vi "Release Session.vi"(6 "force destroy? (F)":bool, 8 "error in":errorcluster, 11 "Session Handle":T1) -> (0 "error out":errorcluster, 3 "file path":path)   [LabVIEW 2015, in "Config Data.lvclass"]
doc: "Release the configuration session for the given reference. If this is the last reference to return, then the config data file will be closed and the file path for the configuration file will be returned."
uses:
  Config Data.lvclass
  Config Session.ctl
  <userlib>/_Session Fwk/Session - Root.lvclass
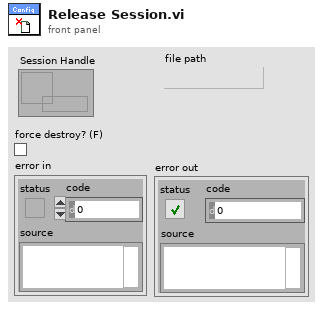
[diagram p1: front panel]
types:
  T1 = typedef "Config Data.lvclass/Config Session.ctl" = refnum<data-value>
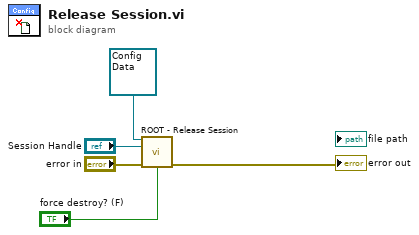
[diagram p0: block diagram]
diagram:
  n1 = call <userlib>:"ROOT - Release Session.vi"("OBJ - Session in"=refnum<class "Config Data.lvclass"> refnum ("Config Data"), "Session Handle in"="Session Handle", "error in (no error)"="error in", "force destroy? (F)"="force destroy? (F)") -> ("error out"=→"error out":errorcluster)  [unwired: 10 in, 1 out]
